vi "check_waypoint.vi"() -> ()   [LabVIEW 2019]
panel:
  in  "wpt cfg":T1={"Waypoint array"=[{"sel"=TRUE, "inv"=FALSE, "path"=path "C:/AGV/Config/waypoint/refwpt_baegot_2course_20201208-3-w-stoppt.txt"}, {"sel"=TRUE, "inv"=TRUE, "path"=path "C:/AGV/Config/waypoint/refwpt_baegot_2course_20201208-3-w-stoppt.txt"}]}
  out "Total map cfg":T2(graph)=[{"ref waypt 0703 A \ngoal point start"=[{"X"=175197.441, "Y"=530326.176}, {"X"=175304.102, "Y"=530277.593}, {"X"=175361.893, "Y"=530247.621}, {"X"=175285.019, "Y"=530145.876}, {"X"=175197.441, "Y"=530326.176}, {"X"=175304.102, "Y"=530277.593}, {"X"=175361.893, "Y"=530247.621}, {"X"=175285.019, "Y"=530145.876}]}, {"ref waypt 0703 A \ngoal point start"=array[12006 elements]}, {"ref waypt 0703 A \ngoal point start"=array[12006 elements]}]
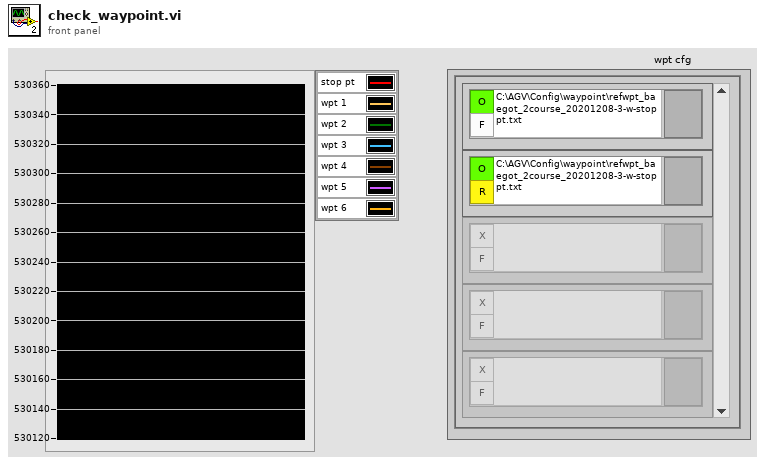
[diagram p1: front panel]
types:
  T1 = cluster{"Waypoint array":cluster{"sel":bool, "inv":bool, "path":path}[]}
  T2 = cluster{"ref waypt 0703 A \ngoal point start":cluster{"X":dbl, "Y":dbl}[]}[]
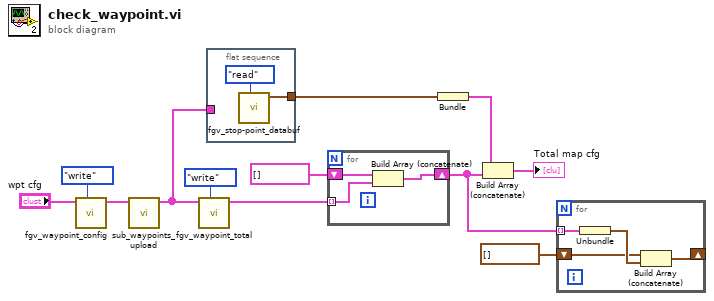
[diagram p0: block diagram]
diagram:
  n1 = call "fgv_waypoint_config.vi"("cmd"=enum16{"read", "write"}."write", "waypoint files cfg"="wpt cfg") -> ("waypoint files cfg out"=w8:T1)  [unwired: 9 in]
  n2 = call "sub_waypoints_upload.vi"("waypoint group"=w8) -> ("waypoint all"=w5:cluster{"XY 그래프":cluster{"X":dbl, "Y":dbl}[]}[])  [unwired: 9 in, 1 out]
  n3 = call "fgv_waypoint_total.vi"("cmd"=enum16{"write", "read"}."write", "waypoint total in"=w5) -> ("waypoint total out"=w4:cluster{"waypt":cluster{"X":dbl, "Y":dbl}[]}[])  [unwired: 9 in]
  n4 = flat-sequence {
    tunnel: [w13] -> w6
    tunnel: w5 -> [_]
    frame #0 {
      n5 = call "fgv_stop-point_databuf.vi"("cmd"=enum16{"clear", "write", "read"}."read") -> ("all stop pts out"=w13:cluster{dbl, dbl}[])  [unwired: 10 in]
    }
  }
  n6 = for {
    shift-right: [w15] -> w2
    shift-left: T2 [] -> [w16]
    tunnel: w4 -> [w17] mode=indexing
    n7 = Build Array (concatenate)(w16, w17) -> (w15:cluster{"waypt":cluster{"X":dbl, "Y":dbl}[]}[])
  }
  n8 = Bundle("all stop pts out"=w6) -> (w3:cluster{"all stop pts out":cluster{dbl, dbl}[]})  [unwired: 1 in]
  n9 = Build Array (concatenate)(w3, w2) -> (→"Total map cfg":T2)
  n10 = for {
    tunnel: w2 -> [w20] mode=indexing
    shift-right: [w21] -> _
    shift-left: cluster{"X":dbl, "Y":dbl}[] [] -> [w18]
    n11 = Unbundle(w20) -> ("ref waypt 0703 A \ngoal point start"=w19:cluster{"X":dbl, "Y":dbl}[])
    n12 = Build Array (concatenate)(w18, w19) -> (w21:cluster{"X":dbl, "Y":dbl}[])
  }
